vi "Reply with Result.vi"(8 "error in (no error)":errorcluster, 10 "Result":refnum<class "Acquired Result.lvclass">, 11 "Result Reply Msg in":refnum<class "Result Reply Msg.lvclass">) -> (0 "error out":errorcluster, 3 "Result Reply Msg out":refnum<class "Result Reply Msg.lvclass">)   [LabVIEW 2016, in "Result Reply Msg.lvclass"]
uses:
  Result Reply Msg.lvclass
  Results/Acquired Result/Acquired Result.lvclass
  Result Reply Msg.lvclass/Result Reply Msg.ctl
  Write Result.vi
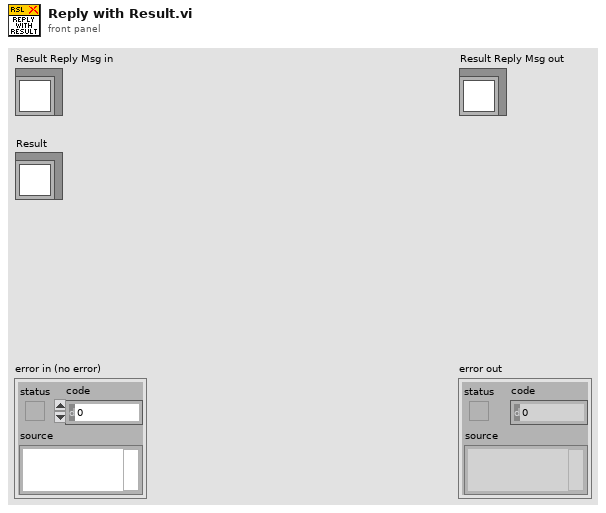
[diagram p1: front panel]
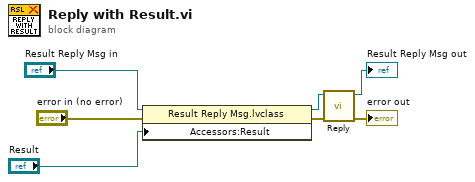
[diagram p0: block diagram]
diagram:
  n1 = property class="Result Reply Msg.lvclass"(reference="Result Reply Msg in", error in="error in (no error)", "Accessors:Result"="Result") -> (reference out=w3:refnum<class "Result Reply Msg.lvclass">, error out=w1:errorcluster)
  n2 = call-dynamic "Reply.vi"("error in (no error)"=w1, "Self-addressed Msg in"=w3) -> ("error out"=→"error out":errorcluster, "Self-addressed Msg out"=→"Result Reply Msg out":refnum<class "Result Reply Msg.lvclass">)  [unwired: 8 in]
